vi "rsidr_core_global.vi"() -> ()   [LabVIEW 2020, in "Rohde&Schwarz RTx Oscilloscopes.lvlib"] (continued)
the indicated waveform.\n\nAvailable Repeated Capabilities:\nNone\n\nRemote-control command(s):\nPOWer:SOA:RESult:TOTal:VIOLation<n>:VOLTage:DATA:YRESolution?"}, {"Level"=6, "Class Only"=TRUE, "Identifier"="", "Descriptive Name"="Current Data", "Data Type"=0, "Command"="", "Access"=0, "Range Table"="", "Read Callback"="", "Write Callback"="", "Supported Models"="", "Instrument Options"="", "Flags"=0, "Help"="Acquires current data."}, {"Level"=6, "Class Only"=TRUE, "Identifier"="", "Descriptive Name"="Current Data Conversion", "Data Type"=0, "Command"="", "Access"=0, "Range Table"="", "Read Callback"="", "Write Callback"="", "Supported Models"="", "Instrument Options"="", "Flags"=0, "Help"="Attributes for conversion of current data."}, {"Level"=7, "Class Only"=FALSE, "Identifier"="RSRTX_ATTR_POWER_SAFE_OPERATING_AREA_RESULT_TOTAL_CURRENT_DATA_CONVERSION_X_START", "Descriptive Name"="Power Safe Operating Area Result Total Current Data Conversion X Start", "Data Type"=1, "Command"="POW:SOA:RES:TOT:VIOL<Point>:CURR:DATA:XOR?", "Access"=0, "Range Table"="", "Read Callback"="rsrtx_FormatSOAPointRepCapReal_ReadCallback.vi", "Write Callback"="", "Supported Models"="RTM|RTA", "Instrument Options"="", "Flags"=0, "Help"="Return the time of the first sample of the indicated waveform.\n\nAvailable Repeated Capabilities:\nNone\n\nRemote-control command(s):\nPOWer:SOA:RESult:TOTal:VIOLation<n>:CURRent:DATA:XORigin?"}, {"Level"=7, "Class Only"=FALSE, "Identifier"="RSRTX_ATTR_POWER_SAFE_OPERATING_AREA_RESULT_TOTAL_CURRENT_DATA_CONVERSION_X_INCREMENT", "Descriptive Name"="Power Safe Operating Area Result Total Current Data Conversion X Increment", "Data Type"=1, "Command"="POW:SOA:RES:TOT:VIOL<Point>:CURR:DATA:XINC?", "Access"=0, "Range Table"="", "Read Callback"="rsrtx_FormatSOAPointRepCapReal_ReadCallback.vi", "Write Callback"="", "Supported Models"="RTM|RTA", "Instrument Options"="", "Flags"=0, "Help"="Return the time difference between two adjacent samples of the indicated waveform.\n\nAvailable Repeated Capabilities:\nNone\n\nRemote-control command(s):\nPOWer:SOA:RESult:TOTal:VIOLation<n>:CURRent:DATA:XINCrement?"}, {"Level"=7, "Class Only"=FALSE, "Identifier"="RSRTX_ATTR_POWER_SAFE_OPERATING_AREA_RESULT_TOTAL_CURRENT_DATA_CONVERSION_Y_START", "Descriptive Name"="Power Safe Operating Area Result Total Current Data Conversion Y Start", "Data Type"=1, "Command"="POW:SOA:RES:TOT:VIOL<Point>:CURR:DATA:YOR?", "Access"=0, "Range Table"="", "Read Callback"="rsrtx_FormatSOAPointRepCapReal_ReadCallback.vi", "Write Callback"="", "Supported Models"="RTM|RTA", "Instrument Options"="", "Flags"=0, "Help"="Return the voltage value for binary value 0 of the indicated waveform.\n\nAvailable Repeated Capabilities:\nNone\n\nRemote-control command(s):\nPOWer:SOA:RESult:TOTal:VIOLation<n>:CURRent:DATA:YORigin?"}, {"Level"=7, "Class Only"=FALSE, "Identifier"="RSRTX_ATTR_POWER_SAFE_OPERATING_AREA_RESULT_TOTAL_CURRENT_DATA_CONVERSION_Y_INCREMENT", "Descriptive Name"="Power Safe Operating Area Result Total Current Data Conversion Y Increment", "Data Type"=1, "Command"="POW:SOA:RES:TOT:VIOL<Point>:CURR:DATA:YINC?", "Access"=0, "Range Table"="", "Read Callback"="rsrtx_FormatSOAPointRepCapReal_ReadCallback.vi", "Write Callback"="", "Supported Models"="RTM|RTA", "Instrument Options"="", "Flags"=0, "Help"="Return the voltage value per bit of the indicated waveform.\n\nAvailable Repeated Capabilities:\nNone\n\nRemote-control command(s):\nPOWer:SOA:RESult:TOTal:VIOLation<n>:CURRent:DATA:YINCrement?"}, {"Level"=7, "Class Only"=FALSE, "Identifier"="RSRTX_ATTR_POWER_SAFE_OPERATING_AREA_RESULT_TOTAL_CURRENT_DATA_CONVERSION_Y_RESOLUTION", "Descriptive Name"="Power Safe Operating Area Result Total Current Data Conversion Y Resolution", "Data Type"=0, "Command"="POW:SOA:RES:TOT:VIOL<Point>:CURR:DATA:YRES?", "Access"=0, "Range Table"="", "Read Callback"="rsrtx_FormatSOAPointRepCapInt_ReadCallback.vi", "Write Callback"="", "Supported Models"="RTM|RTA", "Instrument Options"="", "Flags"=0, "Help"="Return the vertical bit resolution of the indicated waveform.\n\nAvailable Repeated Capabilities:\nNone\n\nRemote-control command(s):\nPOWer:SOA:RESult:TOTal:VIOLation<n>:CURRent:DATA:YRESolution?"}, {"Level"=2, "Class Only"=TRUE, "Identifier"="", "Descriptive Name"="Transient Response", "Data Type"=0, "Command"="", "Access"=0, "Range Table"="", "Read Callback"="", "Write Callback"="", "Supported Models"="", "Instrument Options"="", "Flags"=0, "Help"="Measures the response of a system to a change from equilibrium. This response is described by different properties like the rise time, the overshoot, the settling time, the peak time and the delay time"}, {"Level"=3, "Class Only"=FALSE, "Identifier"="RSRTX_ATTR_START_POWER_TRANSIENT_RESPONSE_MEASUREMENT", "Descriptive Name"="Start Power Transient Response Measurement", "Data Type"=4, "Command"="POW:TRAN:EXEC", "Access"=1, "Range Table"="", "Read Callback"="", "Write Callback"="", "Supported Models"="RTM|RTA", "Instrument Options"="", "Flags"=0, "Help"="Starts the transient response measurement.\n\nAvailable Repeated Capabilities:\nNone\n\nRemote-control command(s):\nPOWer:TRANsient:EXECute"}, {"Level"=3, "Class Only"=FALSE, "Identifier"="RSRTX_ATTR_POWER_TRANSIENT_RESPONSE_SIGNAL_HIGH", "Descriptive Name"="Power Transient Response Signal High", "Data Type"=1, "Command"="POW:TRAN:SIGH", "Access"=2, "Range Table"="rsrtx_rngTransientResponseSignal", "Read Callback"="", "Write Callback"="", "Supported Models"="RTM|RTA", "Instrument Options"="", "Flags"=0, "Help"="Sets the expected signal high voltage value.\n\nAvailable Repeated Capabilities:\nNone\n\nRemote-control command(s):\nPOWer:TRANsient:SIGHigh"}, {"Level"=3, "Class Only"=FALSE, "Identifier"="RSRTX_ATTR_POWER_TRANSIENT_RESPONSE_SIGNAL_LOW", "Descriptive Name"="Power Transient Response Signal Low", "Data Type"=1, "Command"="POW:TRAN:SIGL", "Access"=2, "Range Table"="rsrtx_rngTransientResponseSignal", "Read Callback"="", "Write Callback"="", "Supported Models"="RTM|RTA", "Instrument Options"="", "Flags"=0, "Help"="Sets the expected signal low voltage value.\n\nAvailable Repeated Capabilities:\nNone\n\nRemote-control command(s):\nPOWer:TRANsient:SIGLow"}, {"Level"=3, "Class Only"=FALSE, "Identifier"="RSRTX_ATTR_POWER_TRANSIENT_RESPONSE_ADD_REPORT", "Descriptive Name"="Power Transient Response Add Report", "Data Type"=4, "Command"="POWer:TRANsient:REPort:ADD", "Access"=1, "Range Table"="", "Read Callback"="", "Write Callback"="", "Supported Models"="RTM|RTA", "Instrument Options"="", "Flags"=1, "Help"="Adds the result to the report list.\n\nAvailable Repeated Capabilities:\nNone\n\nRemote-control command(s):\nPOWer:TRANsient:REPort:ADD"}, {"Level"=3, "Class Only"=FALSE, "Identifier"="RSRTX_ATTR_POWER_TRANSIENT_RESPONSE_START_TIME", "Descriptive Name"="Power Transient Response Start Time", "Data Type"=1, "Command"="POW:TRAN:STAR", "Access"=2, "Range Table"="", "Read Callback"="", "Write Callback"="", "Supported Models"="RTM|RTA", "Instrument Options"="", "Flags"=0, "Help"="Sets the start time.\n\nAvailable Repeated Capabilities:\nNone\n\nRemote-control command(s):\nPOWer:TRANsient:STARt"}, {"Level"=3, "Class Only"=FALSE, "Identifier"="RSRTX_ATTR_POWER_TRANSIENT_RESPONSE_STOP_TIME", "Descriptive Name"="Power Transient Response Stop Time", "Data Type"=1, "Command"="POW:TRAN:STOP", "Access"=2, "Range Table"="", "Read Callback"="", "Write Callback"="", "Supported Models"="RTM|RTA", "Instrument Options"="", "Flags"=0, "Help"="Sets the stop time.\n\nAvailable Repeated Capabilities:\nNone\n\nRemote-control command(s):\nPOWer:TRANsient:STOP"}, {"Level"=3, "Class Only"=TRUE, "Identifier"="", "Descriptive Name"="Results", "Data Type"=0, "Command"="", "Access"=0, "Range Table"="", "Read Callback"="", "Write Callback"="", "Supported Models"="", "Instrument Options"="", "Flags"=0, "Help"="Returns transient response results."}, {"Level"=4, "Class Only"=FALSE, "Identifier"="RSRTX_ATTR_POWER_TRANSIENT_RESPONSE_DELAY_TIME", "Descriptive Name"="Power Transient Response Delay Time", "Data Type"=1, "Command"="POW:TRAN:RES:DEL?", "Access"=0, "Range Table"="", "Read Callback"="", "Write Callback"="", "Supported Models"="RTM|RTA", "Instrument Options"="", "Flags"=0, "Help"="Queries the delay time.\n\nAvailable Repeated Capabilities:\nNone\n\nRemote-control command(s):\nPOWer:TRANsient:RESult:DELay?"}, {"Level"=4, "Class Only"=FALSE, "Identifier"="RSRTX_ATTR_POWER_TRANSIENT_RESPONSE_OVERSHOOT", "Descriptive Name"="Power Transient Response Overshoot", "Data Type"=1, "Command"="POW:TRAN:RES:OVER?", "Access"=0, "Range Table"="", "Read Callback"="", "Write Callback"="", "Supported Models"="RTM|RTA", "Instrument Options"="", "Flags"=0, "Help"="Queries the overshoot.\n\nAvailable Repeated Capabilities:\nNone\n\nRemote-control command(s):\nPOWer:TRANsient:RESult:OVERshoot?"}, {"Level"=4, "Class Only"=FALSE, "Identifier"="RSRTX_ATTR_POWER_TRANSIENT_RESPONSE_PEAK_TIME", "Descriptive Name"="Power Transient Response Peak Time", "Data Type"=1, "Command"="POW:TRAN:RES:PEAK:TIME?", "Access"=0, "Range Table"="", "Read Callback"="", "Write Callback"="", "Supported Models"="RTM|RTA", "Instrument Options"="", "Flags"=0, "Help"="Queries the peak time.\n\nAvailable Repeated Capabilities:\nNone\n\nRemote-control command(s):\nPOWer:TRANsient:RESult:PEAK:TIME?"}, {"Level"=4, "Class Only"=FALSE, "Identifier"="RSRTX_ATTR_POWER_TRANSIENT_RESPONSE_PEAK_VALUE", "Descriptive Name"="Power Transient Response Peak Value", "Data Type"=1, "Command"="POW:TRAN:RES:PEAK:VAL?", "Access"=0, "Range Table"="", "Read Callback"="", "Write Callback"="", "Supported Models"="RTM|RTA", "Instrument Options"="", "Flags"=0, "Help"="Queries the peak value.\n\nAvailable Repeated Capabilities:\nNone\n\nRemote-control command(s):\nPOWer:TRANsient:RESult:PEAK:VALue?"}, {"Level"=4, "Class Only"=FALSE, "Identifier"="RSRTX_ATTR_POWER_TRANSIENT_RESPONSE_RISE_TIME", "Descriptive Name"="Power Transient Response Rise Time", "Data Type"=1, "Command"="POW:TRAN:RES:RTIM?", "Access"=0, "Range Table"="", "Read Callback"="", "Write Callback"="", "Supported Models"="RTM|RTA", "Instrument Options"="", "Flags"=0, "Help"="Queries the rise time.\n\nAvailable Repeated Capabilities:\nNone\n\nRemote-control command(s):\nPOWer:TRANsient:RESult:RTIMe?"}, {"Level"=4, "Class Only"=FALSE, "Identifier"="RSRTX_ATTR_POWER_TRANSIENT_RESPONSE_SETTLING_TIME", "Descriptive Name"="Power Transient Response Settling Time", "Data Type"=1, "Command"="POW:TRAN:RES:SETT?", "Access"=0, "Range Table"="", "Read Callback"="", "Write Callback"="", "Supported Models"="RTM|RTA", "Instrument Options"="", "Flags"=0, "Help"="Queries the settling time.\n\nAvailable Repeated Capabilities:\nNone\n\nRemote-control command(s):\nPOWer:TRANsient:RESult:SETTlingtime?"}, {"Level"=1, "Class Only"=TRUE, "Identifier"="", "Descriptive Name"="Spectrum Analysis", "Data Type"=0, "Command"="", "Access"=0, "Range Table"="", "Read Callback"="", "Write Callback"="", "Supported Models"="", "Instrument Options"="", "Flags"=0, "Help"="Contains attributes for Spectrum Analysis."}, {"Level"=2, "Class Only"=FALSE, "Identifier"="RSRTX_ATTR_SPECTRUM_ANALYSIS_ENABLE", "Descriptive Name"="Spectrum Analysis Enable", "Data Type"=3, "Command"="SPEC", "Access"=2, "Range Table"="", "Read Callback"="", "Write Callback"="", "Supported Models"="", "Instrument Options"="", "Flags"=0, "Help"="Switches on the spectrum analysis.\n\nAvailable Repeated Capabilities:\nNone\n\nRemote-control command(s):\nSPECtrum[:STATe]"}, {"Level"=2, "Class Only"=FALSE, "Identifier"="RSRTX_ATTR_SPECTRUM_ANALYSIS_MODE", "Descriptive Name"="Spectrum Analysis Mode", "Data Type"=0, "Command"="SPEC:MODE", "Access"=2, "Range Table"="RsRtx_rngSpectrumAnalysisMode", "Read Callback"="", "Write Callback"="", "Supported Models"="", "Instrument Options"="", "Flags"=0, "Help"="Configures spectrum anaylsis mode.\n\nAvailable Repeated Capabilities:\nNone\n\nRemote-control command(s):\nSPECtrum:MODE"}, {"Level"=2, "Class Only"=FALSE, "Identifier"="RSRTX_ATTR_SPECTRUM_ANALYSIS_SOURCE", "Descriptive Name"="Spectrum Analysis Source", "Data Type"=0, "Command"="SPEC:SOUR", "Access"=2, "Range Table"="rsrtx_rngSource", "Read Callback"="", "Write Callback"="", "Supported Models"="", "Instrument Options"="", "Flags"=0, "Help"="Selects the source for the spectrum analysis diagrams.\n\nAvailable Repeated Capabilities:\nNone\n\nRemote-control command(s):\nSPECtrum:SOURce"}, {"Level"=2, "Class Only"=TRUE, "Identifier"="", "Descriptive Name"="Frequency Domain", "Data Type"=0, "Command"="", "Access"=0, "Range Table"="", "Read Callback"="", "Write Callback"="", "Supported Models"="", "Instrument Options"="", "Flags"=0, "Help"="Contains attributes for Spectrum Frequency Domain."}, {"Level"=3, "Class Only"=FALSE, "Identifier"="RSRTX_ATTR_SPECTRUM_FREQUENCY_AVERAGE_COMPLETE", "Descriptive Name"="Spectrum Frequency Average Complete", "Data Type"=3, "Command"="SPEC:FREQ:AVER:COMP?", "Access"=0, "Range Table"="", "Read Callback"="", "Write Callback"="", "Supported Models"="", "Instrument Options"="", "Flags"=0, "Help"="Returns the state of spectrum averaging.\n\nAvailable Repeated Capabilities:\nNone\n\nRemote-control command(s):\nSPECtrum:FREQuency:AVERage:COMPlete?"}, {"Level"=3, "Class Only"=FALSE, "Identifier"="RSRTX_ATTR_SPECTRUM_FREQUENCY_AVERAGE_COUNT", "Descriptive Name"="Spectrum Frequency Average Count", "Data Type"=0, "Command"="SPEC:FREQ:AVER:COUN", "Access"=2, "Range Table"="", "Read Callback"="", "Write Callback"="", "Supported Models"="", "Instrument Options"="", "Flags"=0, "Help"="Defines the number of spectrums used for averaging.\n\nAvailable Repeated Capabilities:\nNone\n\nRemote-control command(s):\nSPECtrum:FREQuency:AVERage:COUNt"}, {"Level"=3, "Class Only"=FALSE, "Identifier"="RSRTX_ATTR_SPECTRUM_FREQUENCY_MAGNITUDE_SCALE", "Descriptive Name"="Spectrum Frequency Magnitude Scale", "Data Type"=0, "Command"="SPEC:FREQ:MAGN:SCAL", "Access"=2, "Range Table"="RsRtx_rngMagnitudeScale", "Read Callback"="", "Write Callback"="", "Supported Models"="", "Instrument Options"="", "Flags"=0, "Help"="Defines the scaling unit of the y-axis.\n\nAvailable Repeated Capabilities:\nNone\n\nRemote-control command(s):\nSPECtrum:FREQuency:MAGNitude:SCALe"}, {"Level"=3, "Class Only"=FALSE, "Identifier"="RSRTX_ATTR_SPECTRUM_FREQUENCY_POSITION", "Descriptive Name"="Spectrum Frequency Position", "Data Type"=1, "Command"="SPEC:FREQ:POS", "Access"=2, "Range Table"="", "Read Callback"="", "Write Callback"="", "Supported Models"="", "Instrument Options"="", "Flags"=0, "Help"="Defines the position of the spectrum.\n\nAvailable Repeated Capabilities:\nNone\n\nRemote-control command(s):\nSPECtrum:FREQuency:POSition"}, {"Level"=3, "Class Only"=FALSE, "Identifier"="RSRTX_ATTR_SPECTRUM_FREQUENCY_RESET", "Descriptive Name"="Spectrum Frequency Reset", "Data Type"=4, "Command"="SPEC:FREQ:RES", "Access"=1, "Range Table"="", "Read Callback"="", "Write Callback"="", "Supported Models"="", "Instrument Options"="", "Flags"=1, "Help"="Resets the Min, Max and Average waveforms to the current waveform.\n\nAvailable Repeated Capabilities:\nNone\n\nRemote-control command(s):\nSPECtrum:FREQuency:RESet"}, {"Level"=3, "Class Only"=FALSE, "Identifier"="RSRTX_ATTR_SPECTRUM_FREQUENCY_SCALE", "Descriptive Name"="Spectrum Frequency Scale", "Data Type"=1, "Command"="SPEC:FREQ:SCAL", "Access"=2, "Range Table"="", "Read Callback"="", "Write Callback"="", "Supported Models"="", "Instrument Options"="", "Flags"=0, "Help"="Sets the scaling of the spectrum analysis waveform.\n\nAvailable Repeated Capabilities:\nNone\n\nRemote-control command(s):\nSPECtrum:FREQuency:SCALe"}, {"Level"=3, "Class Only"=FALSE, "Identifier"="RSRTX_ATTR_SPECTRUM_FREQUENCY_WINDOW_POSITION", "Descriptive Name"="Spectrum Frequency Window Position", "Data Type"=0, "Command"="DISP:CBAR:FFT", "Access"=2, "Range Table"="", "Read Callback"="", "Write Callback"="", "Supported Models"="", "Instrument Options"="", "Flags"=0, "Help"="Defines the position of the divide bar between normal waveform and FFT window. Sets the vertical position in pixels, measured from the top edge. The vertical display size is 800 px.\n\nAvailable Repeated Capabilities:\nNone\n\nRemote-control command(s):\nDISPlay:CBAR:FFT[:POSition]"}, {"Level"=3, "Class Only"=FALSE, "Identifier"="RSRTX_ATTR_SPECTRUM_FREQUENCY_WINDOW_TYPE", "Descriptive Name"="Spectrum Frequency Window Type", "Data Type"=0, "Command"="SPEC:FREQ:WIND:TYPE", "Access"=2, "Range Table"="RsRtx_rngSpectrumFrequencyWindowType", "Read Callback"="", "Write Callback"="", "Supported Models"="", "Instrument Options"="", "Flags"=0, "Help"="Window functions are multiplied with the input values and thus can improve the spectrum analysis display.\n\nAvailable Repeated Capabilities:\nNone\n\nRemote-control command(s):\nSPECtrum:FREQuency:WINDow:TYPE"}, {"Level"=3, "Class Only"=FALSE, "Identifier"="RSRTX_ATTR_SPECTRUM_FREQUENCY_START", "Descriptive Name"="Spectrum Frequency Start", "Data Type"=1, "Command"="SPEC:FREQ:STAR", "Access"=2, "Range Table"="", "Read Callback"="", "Write Callback"="", "Supported Models"="", "Instrument Options"="", "Flags"=0, "Help"="Defines the start frequency of the displayed frequency domain at the left display edge: Center - Span/2\nYou can set start and stop frequency instead of defining a center frequency and span.\n\nAvailable Repeated Capabilities:\nNone\n\nRemote-control command(s):\nSPECtrum:FREQuency:STARt"}, {"Level"=3, "Class Only"=FALSE, "Identifier"="RSRTX_ATTR_SPECTRUM_FREQUENCY_STOP", "Descriptive Name"="Spectrum Frequency Stop", "Data Type"=1, "Command"="SPEC:FREQ:STOP", "Access"=2, "Range Table"="", "Read Callback"="", "Write Callback"="", "Supported Models"="", "Instrument Options"="", "Flags"=0, "Help"="Defines the stop frequency of the displayed frequency domain at the right display edge: Center + Span/2\nYou can set start and stop frequency instead of defining a center frequency and span.\n\nAvailable Repeated Capabilities:\nNone\n\nRemote-control command(s):\nSPECtrum:FREQuency:STOP"}, {"Level"=3, "Class Only"=FALSE, "Identifier"="RSRTX_ATTR_SPECTRUM_FREQUENCY_CENTER", "Descriptive Name"="Spectrum Frequency Center", "Data Type"=1, "Command"="SPEC:FREQ:CENT", "Access"=2, "Range Table"="", "Read Callback"="", "Write Callback"="", "Supported Models"="", "Instrument Options"="", "Flags"=0, "Help"="Defines the position of the displayed frequency domain, which is (Center - Span/2) to (Center + Span/2). The width of the domain is defined using the command SPECtrum:FREQuency:SPAN.\n\nAvailable Repeated Capabilities:\nNone\n\nRemote-control command(s):\nSPECtrum:FREQuency:CENTer"}, {"Level"=3, "Class Only"=FALSE, "Identifier"="RSRTX_ATTR_SPECTRUM_FREQUENCY_SPAN", "Descriptive Name"="Spectrum Frequency Span", "Data Type"=1, "Command"="SPEC:FREQ:SPAN", "Access"=2, "Range Table"="", "Read Callback"="", "Write Callback"="", "Supported Models"="", "Instrument Options"="", "Flags"=0, "Help"="The span is specified in Hertz and defines the width of the displayed frequency range, which is (Center - Span/2) to (Center + Span/2).\n\nAvailable Repeated Capabilities:\nNone\n\nRemote-control command(s):\nSPECtrum:FREQuency:SPAN"}, {"Level"=3, "Class Only"=FALSE, "Identifier"="RSRTX_ATTR_SPECTRUM_FREQUENCY_FULL_SPAN", "Descriptive Name"="Spectrum Frequency Full Span", "Data Type"=4, "Command"="SPEC:FREQ:FULL", "Access"=1, "Range Table"="", "Read Callback"="", "Write Callback"="", "Supported Models"="", "Instrument Options"="", "Flags"=0, "Help"="Performs the spectrum analysis calculation for the full frequency span.\n\nAvailable Repeated Capabilities:\nNone\n\nRemote-control command(s):\nSPECtrum:FREQuency:FULLspan"}, {"Level"=3, "Class Only"=FALSE, "Identifier"="RSRTX_ATTR_SPECTRUM_FREQUENCY_BANDWIDTH_AUTO", "Descriptive Name"="Spectrum Frequency Bandwidth Auto", "Data Type"=3, "Command"="SPEC:FREQ:BAND:AUTO", "Access"=2, "Range Table"="", "Read Callback"="", "Write Callback"="", "Supported Models"="", "Instrument Options"="", "Flags"=0, "Help"="Enables the auto resolution bandwidth mode. In the auto mode Span:RBW ratio of 1:100 is set.\n\nAvailable Repeated Capabilities:\nNone\n\nRemote-control command(s):\nSPECtrum:FREQuency:BANDwidth[:RESolution]:AUTO"}, {"Level"=3, "Class Only"=FALSE, "Identifier"="RSRTX_ATTR_SPECTRUM_FREQUENCY_BANDWIDTH_RATIO", "Descriptive Name"="Spectrum Frequency Bandwidth Ratio", "Data Type"=1, "Command"="SPEC:FREQ:BAND:RAT", "Access"=2, "Range Table"="", "Read Callback"="", "Write Callback"="", "Supported Models"="", "Instrument Options"="", "Flags"=0, "Help"="Defines the ratio of span (Hz) / resolution bandwidth (Hz). The span/RBW ratio is half the number of points used for FFT which is defined with manual operation in the menu.\n\nAvailable Repeated Capabilities:\nNone\n\nRemote-control command(s):\nSPECtrum:FREQuency:BANDwidth[:RESolution]:RATio"}, {"Level"=3, "Class Only"=FALSE, "Identifier"="RSRTX_ATTR_SPECTRUM_FREQUENCY_BANDWIDTH_RESOLUTION", "Descriptive Name"="Spectrum Frequency Bandwidth Resolution", "Data Type"=1, "Command"="SPEC:FREQ:BAND", "Access"=2, "Range Table"="", "Read Callback"="", "Write Callback"="", "Supported Models"="", "Instrument Options"="", "Flags"=0, "Help"="Defines the resolution bandwidth - the minimum frequency step at which the individual components of a spectrum can be distinguished.\n\nAvailable Repeated Capabilities:\nNone\n\nRemote-control command(s):\nSPECtrum:FREQuency:BANDwidth[:RESolution][:VALue]"}, {"Level"=2, "Class Only"=TRUE, "Identifier"="", "Descriptive Name"="Spectrogram", "Data Type"=0, "Command"="", "Access"=0, "Range Table"="", "Read Callback"="", "Write Callback"="", "Supported Models"="", "Instrument Options"="", "Flags"=0, "Help"="Contains attributes for Spectrogram Settings."}, {"Level"=3, "Class Only"=FALSE, "Identifier"="RSRTX_ATTR_SPECTRUM_SPECTROGRAM_RESET", "Descriptive Name"="Spectrum Spectrogram Reset", "Data Type"=4, "Command"="SPEC:SPEC:RES", "Access"=1, "Range Table"="", "Read Callback"="", "Write Callback"="", "Supported Models"="RTM|RTA", "Instrument Options"="", "Flags"=1, "Help"="Resets the current spectogram and starts a new recording of information.\n\nAvailable Repeated Capabilities:\nNone\n\nRemote-control command(s):\nSPECtrum:SPECtrogram:RESet"}, {"Level"=3, "Class Only"=FALSE, "Identifier"="RSRTX_ATTR_SPECTRUM_SPECTROGRAM_SCALE", "Descriptive Name"="Spectrum Spectrogram Scale", "Data Type"=0, "Command"="SPEC:SPEC:SCAL", "Access"=2, "Range Table"="RsRtx_rngSpectrumSpectrogramScale", "Read Callback"="", "Write Callback"="", "Supported Models"="RTM|RTA", "Instrument Options"="", "Flags"=0, "Help"="Defines a zoom factor for the spectogram.\n\nAvailable Repeated Capabilities:\nNone\n\nRemote-control command(s):\nSPECtrum:SPECtrogram:SCALe"}, {"Level"=3, "Class Only"=FALSE, "Identifier"="RSRTX_ATTR_SPECTRUM_SPECTROGRAM_WINDOW_POSITION", "Descriptive Name"="Spectrum Spectrogram Window Position", "Data Type"=0, "Command"="DISP:CBAR:SPEC", "Access"=2, "Range Table"="", "Read Callback"="", "Write Callback"="", "Supported Models"="", "Instrument Options"="", "Flags"=0, "Help"="Defines the position of the divide bar on top of the spectrogram. Sets the vertical position in pixels, measured from the top edge. The vertical display size is 800 px.\n\nAvailable Repeated Capabilities:\nNone\n\nRemote-control command(s):\nDISPlay:CBAR:SPECtrogram[:POSition]"}, {"Level"=2, "Class Only"=TRUE, "Identifier"="", "Descriptive Name"="Marker", "Data Type"=0, "Command"="", "Access"=0, "Range Table"="", "Read Callback"="", "Write Callback"="", "Supported Models"="", "Instrument Options"="", "Flags"=0, "Help"="Contains attributes for Spectrogram Marker settings."}, {"Level"=3, "Class Only"=FALSE, "Identifier"="RSRTX_ATTR_SPECTRUM_MARKER_ENABLE", "Descriptive Name"="Spectrum Marker Enable", "Data Type"=3, "Command"="SPEC:MARK", "Access"=2, "Range Table"="", "Read Callback"="", "Write Callback"="", "Supported Models"="RTM|RTA", "Instrument Options"="", "Flags"=0, "Help"="Enables the usage of markers.\n\nAvailable Repeated Capabilities:\nNone\n\nRemote-control command(s):\nSPECtrum:MARKer[:ENABle]"}, {"Level"=3, "Class Only"=FALSE, "Identifier"="RSRTX_ATTR_SPECTRUM_MARKER_SOURCE", "Descriptive Name"="Spectrum Marker Source", "Data Type"=0, "Command"="SPEC:MARK:SOUR", "Access"=2, "Range Table"="RsRtx_rngSpectrumMarkerSource", "Read Callback"="", "Write Callback"="", "Supported Models"="RTM|RTA", "Instrument Options"="", "Flags"=0, "Help"="Sets the source for the marker search function.\n\nAvailable Repeated Capabilities:\nNone\n\nRemote-control command(s):\nSPECtrum:MARKer:SOURce"}, {"Level"=3, "Class Only"=FALSE, "Identifier"="RSRTX_ATTR_SPECTRUM_MARKER_DISPLAY", "Descriptive Name"="Spectrum Marker Display", "Data Type"=0, "Command"="SPEC:MARK:DISP", "Access"=2, "Range Table"="RsRtx_rngSpectrumMarkerDisplay", "Read Callback"="", "Write Callback"="", "Supported Models"="RTM|RTA", "Instrument Options"="", "Flags"=0, "Help"="Sets the display settings of the markers on the waveform.\n\nAvailable Repeated Capabilities:\nNone\n\nRemote-control command(s):\nSPECtrum:MARKer:DISPlay"}, {"Level"=3, "Class Only"=FALSE, "Identifier"="RSRTX_ATTR_SPECTRUM_MARKER_SETUP_DISTANCE", "Descriptive Name"="Spectrum Marker Setup Distance", "Data Type"=1, "Command"="SPEC:MARK:SET:DIST", "Access"=2, "Range Table"="", "Read Callback"="", "Write Callback"="", "Supported Models"="RTM|RTA", "Instrument Options"="", "Flags"=0, "Help"="Defines a distance between two subsequent peaks that has to be kept, for the peak to be detected.\n\nAvailable Repeated Capabilities:\nNone\n\nRemote-control command(s):\nSPECtrum:MARKer:SETup:DISTance"}, {"Level"=3, "Class Only"=FALSE, "Identifier"="RSRTX_ATTR_SPECTRUM_MARKER_SETUP_EXCURSION", "Descriptive Name"="Spectrum Marker Setup Excursion", "Data Type"=1, "Command"="SPEC:MARK:SET:EXC", "Access"=2, "Range Table"="", "Read Callback"="", "Write Callback"="", "Supported Models"="RTM|RTA", "Instrument Options"="", "Flags"=0, "Help"="Defines a level deifference between two subsequent peaks that has to be kept, for the peak to be detected.\n\nAvailable Repeated Capabilities:\nNone\n\nRemote-control command(s):\nSPECtrum:MARKer:SETup:EXCursion"}, {"Level"=3, "Class Only"=FALSE, "Identifier"="RSRTX_ATTR_SPECTRUM_MARKER_SETUP_MINIMUM_LEVEL", "Descriptive Name"="Spectrum Marker Setup Minimum Level", "Data Type"=1, "Command"="SPEC:MARK:SET:MLEV", "Access"=2, "Range Table"="", "Read Callback"="", "Write Callback"="", "Supported Models"="RTM|RTA", "Instrument Options"="", "Flags"=0, "Help"="Sets the minimum level for marker peak detection.\n\nAvailable Repeated Capabilities:\nNone\n\nRemote-control command(s):\nSPECtrum:MARKer:SETup:MLEVel"}, {"Level"=3, "Class Only"=FALSE, "Identifier"="RSRTX_ATTR_SPECTRUM_MARKER_SETUP_DETECTION_MODE", "Descriptive Name"="Spectrum Marker Setup Detection Mode", "Data Type"=0, "Command"="SPEC:MARK:SET:MMOD", "Access"=2, "Range Table"="RsRtx_rngSpectrumMarkerSetupDetectionMode", "Read Callback"="", "Write Callback"="", "Supported Models"="RTM|RTA", "Instrument Options"="", "Flags"=0, "Help"="Sets the mode for marker detection.\n\nAvailable Repeated Capabilities:\nNone\n\nRemote-control command(s):\nSPECtrum:MARKer:SETup:MMODe"}, {"Level"=3, "Class Only"=FALSE, "Identifier"="RSRTX_ATTR_SPECTRUM_MARKER_SETUP_MAXIMUM_WIDTH", "Descriptive Name"="Spectrum Marker Setup Maximum Width", "Data Type"=1, "Command"="SPEC:MARK:SET:MWID", "Access"=2, "Range Table"="", "Read Callback"="", "Write Callback"="", "Supported Models"="RTM|RTA", "Instrument Options"="", "Flags"=0, "Help"="Sets the maximum width, that a peak can have for it to be detected.\n\nAvailable Repeated Capabilities:\nNone\n\nRemote-control command(s):\nSPECtrum:MARKer:SETup:MWIDth"}, {"Level"=3, "Class Only"=FALSE, "Identifier"="RSRTX_ATTR_SPECTRUM_MARKER_SETUP_CENTER_SCREEN", "Descriptive Name"="Spectrum Marker Setup Center Screen", "Data Type"=4, "Command"="SPEC:MARK:REF:SET:CSCR", "Access"=1, "Range Table"="", "Read Callback"="", "Write Callback"="", "Supported Models"="RTM|RTA", "Instrument Options"="", "Flags"=0, "Help"="Sets the range to the center of the screen.\n\nAvailable Repeated Capabilities:\nNone\n\nRemote-control command(s):\nSPECtrum:MARKer:REFerence:SETup:CSCReen"}, {"Level"=3, "Class Only"=FALSE, "Identifier"="RSRTX_ATTR_SPECTRUM_MARKER_SETUP_RANGE_TO_PEAK", "Descriptive Name"="Spectrum Marker Setup Range To Peak", "Data Type"=4, "Command"="SPEC:MARK:REF:SET:CMP", "Access"=1, "Range Table"="", "Read Callback"="", "Write Callback"="", "Supported Models"="RTM|RTA", "Instrument Options"="", "Flags"=0, "Help"="Sets the range to the highest peak.\n\nAvailable Repeated Capabilities:\nNone\n\nRemote-control command(s):\nSPECtrum:MARKer:REFerence:SETup:CMPeak"}, {"Level"=3, "Class Only"=FALSE, "Identifier"="RSRTX_ATTR_SPECTRUM_MARKER_REFERENCE_MODE", "Descriptive Name"="Spectrum Marker Reference Mode", "Data Type"=0, "Command"="SPEC:MARK:REF:SET:MODE", "Access"=2, "Range Table"="RsRtx_rngSpectrumMarkerReferenceMode", "Read Callback"="", "Write Callback"="", "Supported Models"="RTM|RTA", "Instrument Options"="", "Flags"=0, "Help"="Sets the mode for the selection of the reference peak. The peak with the highest level within the selected settings is set as the reference marker.\n\nAvailable Repeated Capabilities:\nNone\n\nRemote-control command(s):\nSPECtrum:MARKer:REFerence:SETup:MODE"}, {"Level"=3, "Class Only"=FALSE, "Identifier"="RSRTX_ATTR_SPECTRUM_MARKER_REFERENCE_FREQUENCY", "Descriptive Name"="Spectrum Marker Reference Frequency", "Data Type"=1, "Command"="SPEC:MARK:REF:SET:FREQ", "Access"=2, "Range Table"="", "Read Callback"="", "Write Callback"="", "Supported Models"="RTM|RTA", "Instrument Options"="", "Flags"=0, "Help"="Sets the center frequency for the capture range, when SPECtrum:MARKer:REFerence:SETup:MODE RANGe.\n\nAvailable Repeated Capabilities:\nNone\n\nRemote-control command(s):\nSPECtrum:MARKer:REFerence:SETup:FREQuency"}, {"Level"=3, "Class Only"=FALSE, "Identifier"="RSRTX_ATTR_SPECTRUM_MARKER_REFERENCE_SPAN", "Descriptive Name"="Spectrum Marker Reference Span", "Data Type"=1, "Command"="SPEC:MARK:REF:SET:SPAN", "Access"=2, "Range Table"="", "Read Callback"="", "Write Callback"="", "Supported Models"="RTM|RTA", "Instrument Options"="", "Flags"=0, "Help"="Sets the span range, which is defined as the ratio of the capture range and the width of the specified reference mode, when SPECtrum:MARKer:REFerence:SETup:MODE RANGe.\n\nAvailable Repeated Capabilities:\nNone\n\nRemote-control command(s):\nSPECtrum:MARKer:REFerence:SETup:SPAN"}, {"Level"=3, "Class Only"=FALSE, "Identifier"="RSRTX_ATTR_SPECTRUM_MARKER_REFERENCE_INDEX", "Descriptive Name"="Spectrum Marker Reference Index", "Data Type"=0, "Command"="SPEC:MARK:REF:SET:IND", "Access"=2, "Range Table"="", "Read Callback"="", "Write Callback"="", "Supported Models"="RTM|RTA", "Instrument Options"="", "Flags"=0, "Help"="Sets the reference marker to the peak with the specified index, when SPECtrum:MARKer:REFerence:SETup:MODE INDicated.\n\nAvailable Repeated Capabilities:\nNone\n\nRemote-control command(s):\nSPECtrum:MARKer:REFerence:SETup:INDex"}, {"Level"=3, "Class Only"=TRUE, "Identifier"="", "Descriptive Name"="Spectrum Marker Table", "Data Type"=0, "Command"="", "Access"=0, "Range Table"="", "Read Callback"="", "Write Callback"="", "Supported Models"="", "Instrument Options"="", "Flags"=0, "Help"="Contains attributes for Marker Table Settings."}, {"Level"=4, "Class Only"=FALSE, "Identifier"="RSRTX_ATTR_SPECTRUM_MARKER_TABLE_ENABLE", "Descriptive Name"="Spectrum Marker Table Enable", "Data Type"=3, "Command"="SPEC:MARK:RTAB:ENAB", "Access"=2, "Range Table"="", "Read Callback"="", "Write Callback"="", "Supported Models"="RTM|RTA", "Instrument Options"="", "Flags"=0, "Help"="Enables the display of the marker table.\n\nAvailable Repeated Capabilities:\nNone\n\nRemote-control command(s):\nSPECtrum:MARKer:RTABle:ENABle"}, {"Level"=4, "Class Only"=FALSE, "Identifier"="RSRTX_ATTR_SPECTRUM_MARKER_TABLE_DETECTED_PEAKS", "Descriptive Name"="Spectrum Marker Table Detected Peaks", "Data Type"=0, "Command"="SPEC:MARK:RCO?", "Access"=0, "Range Table"="", "Read Callback"="", "Write Callback"="", "Supported Models"="RTM|RTA", "Instrument Options"="", "Flags"=0, "Help"="Returns the number of detected peaks.\n\nAvailable Repeated Capabilities:\nNone\n\nRemote-control command(s):\nSPECtrum:MARKer:RCOunt?"}, {"Level"=4, "Class Only"=FALSE, "Identifier"="RSRTX_ATTR_SPECTRUM_MARKER_TABLE_RESULT_MODE", "Descriptive Name"="Spectrum Marker Table Result Mode", "Data Type"=0, "Command"="SPEC:MARK:RMOD", "Access"=2, "Range Table"="RsRtx_rngSpectrumMarkerResultMode", "Read Callback"="", "Write Callback"="", "Supported Models"="RTM|RTA", "Instrument Options"="", "Flags"=0, "Help"="Sets the mode for the display of the results in the marker table.\n\nAvailable Repeated Capabilities:\nNone\n\nRemote-control command(s):\nSPECtrum:MARKer:RMODe"}, {"Level"=4, "Class Only"=FALSE, "Identifier"="RSRTX_ATTR_SPECTRUM_MARKER_TABLE_POSITION", "Descriptive Name"="Spectrum Marker Table Position", "Data Type"=0, "Command"="SPEC:MARK:RTAB:POS", "Access"=2, "Range Table"="RsRtx_rngSpectrumMarkerTablePosition", "Read Callback"="", "Write Callback"="", "Supported Models"="RTM|RTA", "Instrument Options"="", "Flags"=0, "Help"="Defines the position of the marker table on the screen: top right, bottom right, or full screen. With full screen setting, the table covers nearly the complete righthand half of the screen.\n\nAvailable Repeated Capabilities:\nNone\n\nRemote-control command(s):\nSPECtrum:MARKer:RTABle:POSition"}, {"Level"=3, "Class Only"=TRUE, "Identifier"="", "Descriptive Name"="Results", "Data Type"=0, "Command"="", "Access"=0, "Range Table"="", "Read Callback"="", "Write Callback"="", "Supported Models"="", "Instrument Options"="", "Flags"=0, "Help"="The result values include the result number ant the corresponding frequency and magnitude."}, {"Level"=4, "Class Only"=FALSE, "Identifier"="RSRTX_ATTR_SPECTRUM_REFERENCE_MARKER_FREQUENCY", "Descriptive Name"="Spectrum Reference Marker Frequency", "Data Type"=1, "Command"="SPEC:MARK:RMAR:FREQ?", "Access"=0, "Range Table"="", "Read Callback"="", "Write Callback"="", "Supported Models"="", "Instrument Options"="", "Flags"=0, "Help"="Returns the frequency of the reference marker.\n\nAvailable Repeated Capabilities:\nNone\n\nRemote-control command(s):\nSPECtrum:MARKer:RMARker:FREQuency?"}, {"Level"=4, "Class Only"=FALSE, "Identifier"="RSRTX_ATTR_SPECTRUM_REFERENCE_MARKER_LEVEL", "Descriptive Name"="Spectrum Reference Marker Level", "Data Type"=1, "Command"="SPEC:MARK:RMAR:LEV?", "Access"=0, "Range Table"="", "Read Callback"="", "Write Callback"="", "Supported Models"="", "Instrument Options"="", "Flags"=0, "Help"="Returns the level of the reference marker.\n\nAvailable Repeated Capabilities:\nNone\n\nRemote-control command(s):\nSPECtrum:MARKer:RMARker:LEVel?"}, {"Level"=2, "Class Only"=TRUE, "Identifier"="", "Descriptive Name"="Display", "Data Type"=0, "Command"="", "Access"=0, "Range Table"="", "Read Callback"="", "Write Callback"="", "Supported Models"="", "Instrument Options"="", "Flags"=0, "Help"="Contains attributes for Spectrogram Diagram Display Settings."}, {"Level"=3, "Class Only"=FALSE, "Identifier"="RSRTX_ATTR_SPECTRUM_DISPLAY_MAGNITUDE_MODE", "Descriptive Name"="Spectrum Display Magnitude Mode", "Data Type"=3, "Command"="SPEC:DIAG:COL:MAGN:MODE", "Access"=2, "Range Table"="", "Read Callback"="", "Write Callback"="", "Supported Models"="RTM|RTA", "Instrument Options"="", "Flags"=0, "Help"="Enables the magnitude coloring of the waveform.\n\nAvailable Repeated Capabilities:\nNone\n\nRemote-control command(s):\nSPECtrum:DIAGram:COLor:MAGNitude:MODE"}, {"Level"=3, "Class Only"=FALSE, "Identifier"="RSRTX_ATTR_SPECTRUM_DISPLAY_MAXIMUM_LEVEL", "Descriptive Name"="Spectrum Display Maximum Level", "Data Type"=1, "Command"="SPEC:DIAG:COL:MAX", "Access"=2, "Range Table"="", "Read Callback"="", "Write Callback"="", "Supported Models"="RTM|RTA", "Instrument Options"="", "Flags"=0, "Help"="Sets the level used as a maximum for the color scale selected with SPECtrum:DIAGram:COLor:SCHeme:FDOMain/SPECtrum:DIAGram:COLor:SCHeme:SPECtrogramm . All level values higher than the maximum will be displayed with the maximum color.\n\nAvailable Repeated Capabilities:\nNone\n\nRemote-control command(s):\nSPECtrum:DIAGram:COLor:MAXimum[:LEVel]"}, {"Level"=3, "Class Only"=FALSE, "Identifier"="RSRTX_ATTR_SPECTRUM_DISPLAY_MINIMUM_LEVEL", "Descriptive Name"="Spectrum Display Minimum Level", "Data Type"=1, "Command"="SPEC:DIAG:COL:MIN", "Access"=2, "Range Table"="", "Read Callback"="", "Write Callback"="", "Supported Models"="RTM|RTA", "Instrument Options"="", "Flags"=0, "Help"="Sets the level used as a minimum of the color scale selected with SPECtrum:DIAGram:COLor:SCHeme:FDOMain/SPECtrum:DIAGram:COLor:SCHeme:SPECtrogramm. All level values lower than the minimum will be displayed with the minimum color.\n\nAvailable Repeated Capabilities:\nNone\n\nRemote-control command(s):\nSPECtrum:DIAGram:COLor:MINimum[:LEVel]"}, {"Level"=3, "Class Only"=FALSE, "Identifier"="RSRTX_ATTR_SPECTRUM_DISPLAY_COLOR_SCHEME", "Descriptive Name"="Spectrum Display Color Scheme", "Data Type"=0, "Command"="SPEC:DIAG:COL:SCH:FDOM", "Access"=2, "Range Table"="RsRtx_rngSpectrumDisplayColorScheme", "Read Callback"="", "Write Callback"="", "Supported Models"="RTM|RTA", "Instrument Options"="", "Flags"=0, "Help"="Sets the color scale for the display of the waveform in the frequency domain diagram.\n\nAvailable Repeated Capabilities:\nNone\n\nRemote-control command(s):\nSPECtrum:DIAGram:COLor:SCHeme:FDOMain"}, {"Level"=3, "Class Only"=FALSE, "Identifier"="RSRTX_ATTR_SPECTRUM_DISPLAY_SPECTROGRAM_COLOR_SCHEME", "Descriptive Name"="Spectrum Display Spectrogram Color Scheme", "Data Type"=0, "Command"="SPEC:DIAG:COL:SCH:SPEC", "Access"=2, "Range Table"="RsRtx_rngSpectrumDisplayColorScheme", "Read Callback"="", "Write Callback"="", "Supported Models"="RTM|RTA", "Instrument Options"="", "Flags"=0, "Help"="Sets the color scale for the display of the spectogram.\n\nAvailable Repeated Capabilities:\nNone\n\nRemote-control command(s):\nSPECtrum:DIAGram:COLor:SCHeme:SPECtrogramm"}, {"Level"=3, "Class Only"=FALSE, "Identifier"="RSRTX_ATTR_SPECTRUM_DISPLAY_FREQUENCY_DOMAIN_ENABLE", "Descriptive Name"="Spectrum Display Frequency Domain Enable", "Data Type"=3, "Command"="SPEC:DIAG:FDOM", "Access"=2, "Range Table"="", "Read Callback"="", "Write Callback"="", "Supported Models"="RTM|RTA", "Instrument Options"="", "Flags"=0, "Help"="Enables the display of the frequency domain diagram.\n\nAvailable Repeated Capabilities:\nNone\n\nRemote-control command(s):\nSPECtrum:DIAGram:FDOMain[:ENABle]"}, {"Level"=3, "Class Only"=FALSE, "Identifier"="RSRTX_ATTR_SPECTRUM_DISPLAY_SPECTROGRAM_ENABLE", "Descriptive Name"="Spectrum Display Spectrogram Enable", "Data Type"=3, "Command"="SPEC:DIAG:SPEC", "Access"=2, "Range Table"="", "Read Callback"="", "Write Callback"="", "Supported Models"="RTM|RTA", "Instrument Options"="", "Flags"=0, "Help"="Enables the display of the spectrum diagram.\n\nAvailable Repeated Capabilities:\nNone\n\nRemote-control command(s):\nSPECtrum:DIAGram:SPECtrogram[:ENABle]"}, {"Level"=3, "Class Only"=FALSE, "Identifier"="RSRTX_ATTR_SPECTRUM_DISPLAY_TIME_DOMAIN_ENABLE", "Descriptive Name"="Spectrum Display Time Domain Enable", "Data Type"=3, "Command"="SPEC:DIAG:TDOM", "Access"=2, "Range Table"="", "Read Callback"="", "Write Callback"="", "Supported Models"="RTM|RTA", "Instrument Options"="", "Flags"=0, "Help"="Enables the display of the time domain diagram.\n\nAvailable Repeated Capabilities:\nNone\n\nRemote-control command(s):\nSPECtrum:DIAGram:TDOMain[:ENABle]"}, {"Level"=2, "Class Only"=TRUE, "Identifier"="", "Descriptive Name"="Waveform", "Data Type"=0, "Command"="", "Access"=0, "Range Table"="", "Read Callback"="", "Write Callback"="", "Supported Models"="", "Instrument Options"="", 
